vi "Make Protection Signal.vi"(11 "Node Ptr":T1=18446744073709551615 format="%.0x") -> ()   [LabVIEW 2015, in "Protection and Counter Addon System Explorer.lvlib"]
uses:
  Protection and Counter Addon System Explorer.lvlib
  <vilib>/NI Veristand/Custom Device API/Custom Device Item Ref.ctl
  Shared/SubVIs/GUID Lookup.vi
  Shared/Protection and Counter Addon Shared.lvlib
  SubModules/Frame Protection Support/Source/System Explorer/Protection and Counter Support System Explorer.lvlib
  <vilib>/NI VeriStand/Custom Device API/Custom Device API.lvlib
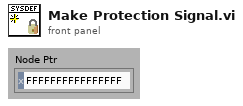
[diagram p1: front panel]
types:
  T1 = typedef "Custom Device API.lvlib/Custom Device Item Ref.ctl" = u64
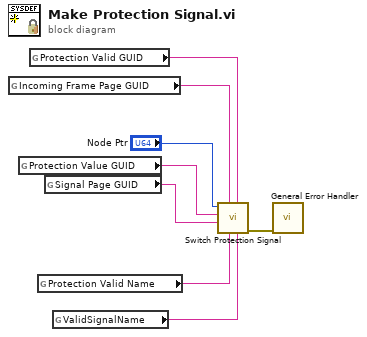
[diagram p0: block diagram]
diagram:
  n1 = global read "GUID Lookup.vi" "Incoming Frame Page GUID"() -> (w3:string)
  n2 = global read "GUID Lookup.vi" "Protection Value GUID"() -> (w6:string)
  n3 = global read "GUID Lookup.vi" "Protection Valid GUID"() -> (w2:string)
  n4 = global read "GUID Lookup.vi" "Protection Valid Name"() -> (w4:string)
  n5 = global read "GUID Lookup.vi" "Signal Page GUID"() -> (w5:string)
  n6 = global read "GUID Lookup.vi" "ValidSignalName"() -> (w1:string)
  n7 = call "Switch Protection Signal.vi"("Valid Signal Name"=w1, "Protection Valid GUID"=w2, "Protection Valid Name"=w4, "Incoming Frame GUID"=w3, "Signal Page GUID"=w5, "Protection Value GUID"=w6, "Node Ptr"="Node Ptr") -> ("error out"=w8:errorcluster)  [unwired: 4 in]
  n8 = call <vilib>:"General Error Handler.vi"("error in (no error)"=w8) -> ()  [unwired: 10 in, 5 out]
